vi "Load Plugin.vi"(6 "timeout (ms)":i32=5000, 8 "error in":errorcluster, 10 "New Plugin":T1, 11 "gRPC ID in":T2) -> (0 "error out":errorcluster, 3 "gRPC ID out":T2)   [LabVIEW 2021, in "CIFManagerClientWrapper.lvlib"]
uses:
  CIFManagerClientWrapper.lvlib
  <vilib>/gRPC/LabVIEW gRPC Library/Shared/grpcId.ctl
  typedefs/New Plugin.ctl
  CIF_Manager_client/RPC Messages/cif_manager_LoadPluginRequest.ctl
  CIF_Manager_client/CIF_Manager_client.lvlib
  <vilib>/gRPC/LabVIEW gRPC Library/grpc-lvsupport-release.lvlib
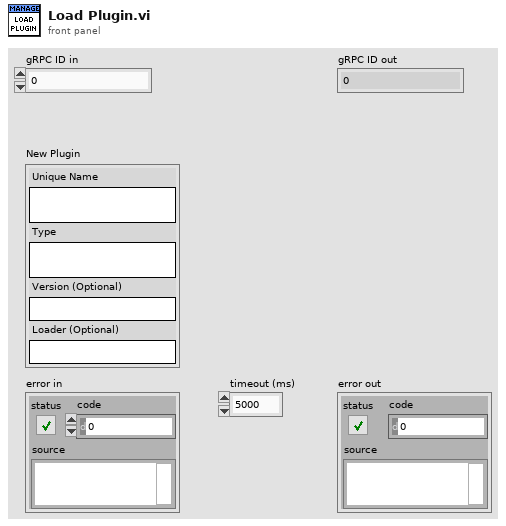
[diagram p1: front panel]
types:
  T1 = typedef "CIFManagerClientWrapper.lvlib/New Plugin.ctl" = cluster{"Unique Name":string, "Type":string, "Version (Optional)":string, "Loader (Optional)":string}
  T2 = typedef "grpc-lvsupport-release.lvlib/grpcId.ctl" = u64
  T3 = typedef "CIF_Manager_client.lvlib/cif_manager_LoadPluginRequest.ctl" = cluster{"plugin_type":string, "plugin_name":string, "version":string, "loader_process":string}
  T4 = typedef "CIF_Manager_client.lvlib/cif_manager_LoadPluginResponse.ctl" = cluster{"status":T5}
  T5 = typedef "CIF_Manager_client.lvlib/cif_common_Status.ctl" = cluster{"code":i32, "message":string}
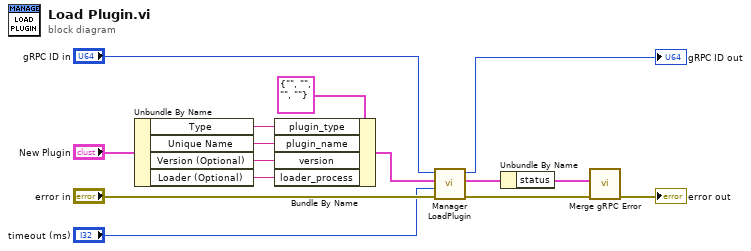
[diagram p0: block diagram]
diagram:
  n1 = Unbundle By Name("New Plugin") -> ("Type"=w6:string, "Unique Name"=w5:string, "Version (Optional)"=w4:string, "Loader (Optional)"=w3:string)
  n2 = Bundle By Name(cluster=T3 {"plugin_type"="", "plugin_name"="", "version"="", "loader_process"=""} ("Request Data"), "plugin_type"=w6, "plugin_name"=w5, "version"=w4, "loader_process"=w3) -> (w8:T3)
  n3 = call "Manager LoadPlugin.vi"("error in"="error in", "timeout (ms)"="timeout (ms)", "Request Data"=w8, "gRPC ID"="gRPC ID in") -> ("error out"=w11:errorcluster, "Response Data"=w9:T4, "gRPC ID out"=→"gRPC ID out":T2)  [unwired: 5 in]
  n4 = Unbundle By Name(w9) -> ("status"=w1:T5)
  n5 = call "Merge gRPC Error.vi"("error in (no error)"=w11, "gRPC Error"=w1) -> ("error out"=→"error out":errorcluster)  [unwired: 9 in]
